vi "CRYVirtual Window.vi"   [LabVIEW 2013]
uses:
  SubVI/CRYMain Sub Window Global.vi
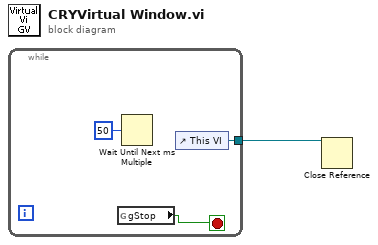
[diagram p0: block diagram]
diagram:
  n1 = while {
    tunnel: [w2] -> w1
    stop <- w3 stop-if-true
    n2 = global read "CRYMain Sub Window Global.vi" "gStop"() -> (w3:bool)
    n3 = Wait Until Next ms Multiple(millisecond multiple=u32 50) -> ()  [unwired: 1 out]
    n4 = control-ref of="This VI"() -> (w2:refnum<vi>)
  }
  n5 = Close Reference(reference=w1) -> ()  [unwired: 1 in, 1 out]
